vi "MHM Read Register.vi"(8 "error in (no error)":errorcluster, 9 "pulNumberOfBytes":u32, 10 "ulAdr":u32, 11 "ulMHMHandle":u32) -> (0 "error out":errorcluster, 1 "pulData":u32[](array[numeric]), 2 "pulNumberOfBytes out":u32, 3 "function return":u32)   [LabVIEW 2017, in "MHM_1SL_interface.lvlib"]
uses:
  MHM_1SL_interface.lvlib
  SSI_Tool/DUT_Interface/lv_interface/lib/MHM_1SL_interface.dll
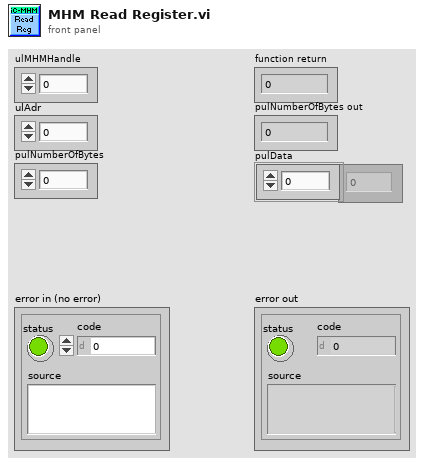
[diagram p1: front panel]
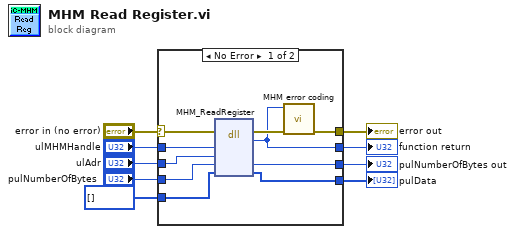
[diagram p0: block diagram]
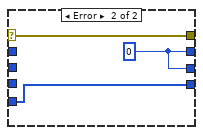
[diagram p2: hidden frame]
diagram:
  n1 = case shown="No Error" "error in (no error)" {
    selector: "error in (no error)" -> [w19 w22]
    tunnel: "ulMHMHandle" -> [w18 _]
    tunnel: [w16 w22] -> w7
    tunnel: [w15 w20] -> w6
    tunnel: "ulAdr" -> [w14 _]
    tunnel: "pulNumberOfBytes" -> [w13 _]
    tunnel: [w12 w20] -> w3
    tunnel: [w11 w21] -> w2
    tunnel: u32[] [] ("pulData") -> [w10 w21]
    frame No Error {
      n2 = dll-call lib="C:/workspace/project/scancon/sw/SSI_Tool/DUT_Interface/lv_interface/lib/MHM_1SL_interface.dll" fn="MHM_ReadRegister"(error in=w19, "ulMHMHandle"=w18, "ulAdr"=w14, "pulNumberOfBytes"=w13, "pulData"=w10) -> (error out=w17:errorcluster, "return type"=w15:u32, "pulNumberOfBytes"=w12:u32, "pulData"=w11:u32[])  [unwired: 4 in, 1 out]
      n3 = call "MHM error coding.vi"("error in (no error)"=w17, "function return in"=w15) -> ("error out"=w16:errorcluster)  [unwired: 9 in]
    }
    frame Error {
      w20 = u32 0 ("return type")
    }
  }
  "function return" <- w6
  "error out" <- w7
  "pulNumberOfBytes out" <- w3
  "pulData" <- w2
